vi "Apply VNS to Random Solution.vi"(7 "Max Allowed Time Passed?":bool, 8 "error in (no error)":errorcluster, 10 "GA in":refnum<class "GA.lvclass">, 11 "OSSP_Problem in":refnum<class "OSSP_Problem.lvclass">) -> (0 "error out":errorcluster, 2 "GA out":refnum<class "GA.lvclass">, 3 "OSSP_Problem out":refnum<class "OSSP_Problem.lvclass">)   [LabVIEW 2013]
uses:
  Classes/GA.lvclass
  Classes/OSSP_Problem.lvclass
  Classes/GA.lvclass/GA.ctl
  Classes/OSSP_Problem.lvclass/OSSP_Problem.ctl
  Classes/GA_Class/Controls/Solution_GA.ctl
  Insert Neighborhood.vi
  Inversion Neighborhood.vi
  Zobolas Local Search Engine.vi
  Classes/OSSP_Problem_Class/Getters/Read Number of Machines.vi
  VNS Zobolas LSA Scheduler Selector.vi
  GA/SubVIS/Remove Duplicates In Array.vi
  Generate Two Indices for Local Search.vi
  Or-Opt(Zobolas) Neighborhood.vi
  Swap Neighborhood.vi
  Classes/Scheduler_Class/Prins FIFO Scheduler Methods and Controls/Methods/Calculate Makespan (Prins FIFO Engine).vi
  Classes/Scheduler_Class/Prins FIFO Scheduler Methods and Controls/Methods/Calculate Tardiness (Prins FIFO Engine).vi
  Classes/Scheduler_Class/NonDelay Scheduler/Non Delay Scheduler Engine.vi
  Classes/OSSP_Problem_Class/Getters/Read Number of Jobs.vi
  Classes/OSSP_Problem_Class/Getters/Read Processing Times.vi
  GA/SubVIS/Calcualte General Tardiness.vi
  Classes/OSSP_Problem_Class/Getters/Read Due Dates.vi
  Classes/Scheduler_Class/Giffler Thompson Active Schedule Engine.vi
  Classes/Scheduler_Class/Prins FIFO Scheduler Methods and Controls/Prins FIFO Scheduler.vi
  Classes/Scheduler_Class/Prins FIFO Scheduler Methods and Controls/Methods/Calculate Final Completion Times of Jobs.vi
  Classes/Scheduler_Class/Prins FIFO Scheduler Methods and Controls/Methods/Reorder Schedule(Prins FIFO) based on Start Times.vi
  Classes/Scheduler_Class/Operation to Machine Job Tuple.vi
  Classes/Scheduler_Class/Prins FIFO Scheduler Methods and Controls/Methods/UpdateMachineGaps.vi
  Classes/Scheduler_Class/Prins FIFO Scheduler Methods and Controls/Methods/UpdateJobGaps.vi
  Classes/Scheduler_Class/Prins FIFO Scheduler Methods and Controls/Methods/Find Intersecting Gaps.vi
  Classes/Scheduler_Class/GT Algorithm Find M_ok and J_ok.vi
  Classes/Scheduler_Class/Prins FIFO Scheduler Methods and Controls/Methods/Transform to Plain Job and Machine Gaps Array.vi
  Classes/Scheduler_Class/Semiactive Scheduler/Semi Active Scheduler Engine.vi
  Nonredundant Swap Neighborhood.vi
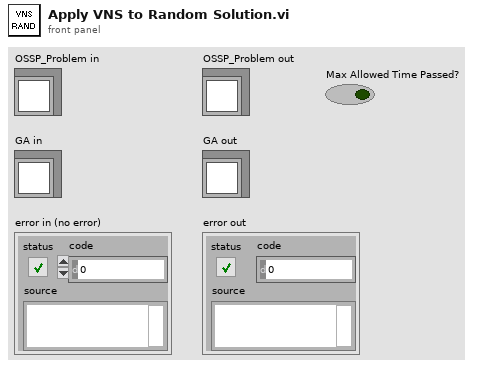
[diagram p1: front panel]
types:
  T1 = typedef "Solution_GA.ctl" = cluster{"Schedule":u16[], "Fitness":u16, "Fitness Valid?":bool}
  T2 = typedef "Objective.ctl" = enum16{"Makespan", "Total Tardiness"}
  T3 = typedef "Scheduler Type.ctl" = enum16{"Non Delay Scheduler", "GT Active Scheduler", "My Faulty Scheduler", "Prins FIFO Scheduler", "SemiActive Scheduler"}
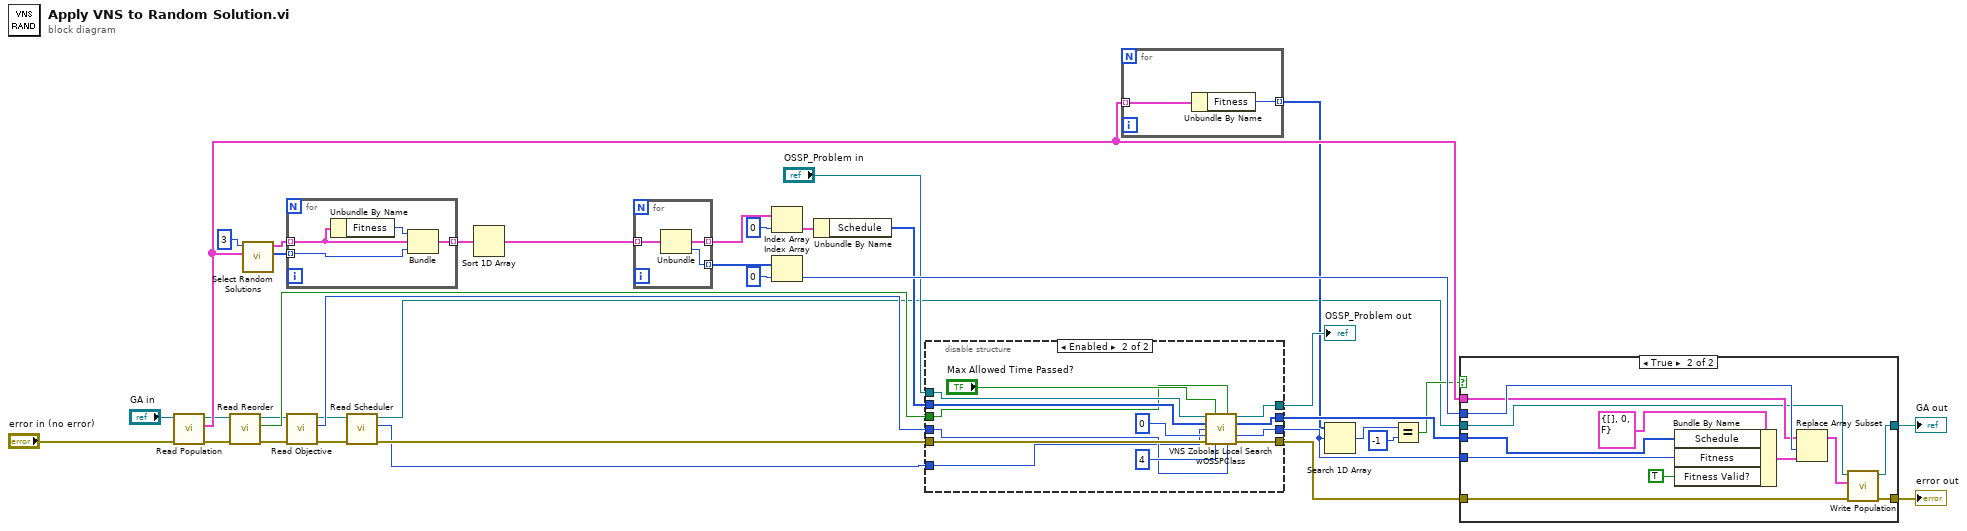
[diagram p0: block diagram]
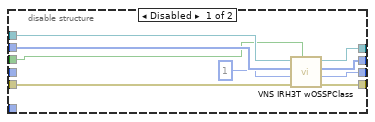
[diagram p3: hidden frame]
diagram:
  n1 = call "Read Population.vi"("error in (no error)"="error in (no error)", "GA in"="GA in") -> ("error out"=w12:errorcluster, "Population"=w20:T1[], "GA out"=w11:refnum<class "GA.lvclass">)  [unwired: 7 in]
  n2 = call "Read Reorder.vi"("error in (no error)"=w12, "GA in"=w11) -> ("error out"=w8:errorcluster, "Reorder"=w10:bool, "GA out"=w7:refnum<class "GA.lvclass">)  [unwired: 7 in]
  n3 = call "Select Random Solutions.vi"("Population"=w20, "Tournament Size"=3) -> ("Solution Indices"=w27:i32[], "Selected Solutions"=w31:T1[])  [unwired: 8 in]
  n4 = for {
    tunnel: w31 -> [w40] mode=indexing
    tunnel: [w39] -> w30 mode=indexing
    tunnel: w27 -> [w38] mode=indexing
    n5 = Unbundle By Name(w40) -> ("Fitness"=w41:u16)
    n6 = Bundle("Fitness"=w41, "Solution"=w40, w38) -> (w39:cluster{"Fitness":u16, "Solution":T1, i32})  [unwired: 1 in]
  }
  n7 = call "Read Objective .vi"("error in (no error)"=w8, "GA in"=w7) -> ("error out"=w3:errorcluster, "Objective"=w6:T2, "GA out"=w5:refnum<class "GA.lvclass">)  [unwired: 7 in]
  n8 = call "Read Scheduler.vi"("error in (no error)"=w3, "GA in"=w5) -> ("error out"=w2:errorcluster, "Scheduler"=w1:T3, "GA out"=w4:refnum<class "GA.lvclass">)  [unwired: 7 in]
  n9 = Sort 1D Array(array=w30) -> (sorted array=w21:cluster{"Fitness":u16, "Solution":T1, i32}[])
  n10 = for {
    tunnel: w21 -> [w44] mode=indexing
    tunnel: [w43] -> w29 mode=indexing
    tunnel: [w42] -> w26 mode=indexing
    n11 = Unbundle(w44) -> ("Solution"=w43:T1, w42:i32)  [unwired: 1 out]
  }
  n12 = Index Array(array=w29, index=0) -> (element=w24:T1)
  n13 = Index Array(array=w26, index=0) -> (element=w22:i32)
  n14 = Unbundle By Name(w24) -> ("Schedule"=w15:u16[])
  n15 = disable-structure shown="Enabled" {
    disable-tunnel: [w53 w65] -> w33
    disable-tunnel: [w52 w59] -> w23
    disable-tunnel: [w51 w61] -> w17
    disable-tunnel: [w50 w62] -> w16
    disable-tunnel: w15 -> [w49 w64]
    disable-tunnel: "OSSP_Problem in" -> [w48 w66]
    disable-tunnel: w2 -> [w46 w60]
    disable-tunnel: w10 -> [w45 w56]
    disable-tunnel: w6 -> [_ w55]
    disable-tunnel: w1 -> [_ w54]
    frame Disabled {
      n16 = call "VNS IRH3T wOSSPClass.vi"("Reorder?"=w45, "error in (no error)"=w46, "Max Iteration Count"=1, "Best Chromosome In"=w49, "OSSP_Problem.lvclass"=w48) -> ("error out"=w52:errorcluster, "Tardiness(FIFO Engine)"=w51:u16, "VNS Result"=w50:u16[], "OSSP_Problem out"=w53:refnum<class "OSSP_Problem.lvclass">)  [unwired: 3 in]
    }
    frame Enabled {
      n17 = call "VNS Zobolas Local Search wOSSPClass.vi"("OSSP_Problem.lvclass"=w66, "Max Allowed Time Passed?"="Max Allowed Time Passed?", "Reorder?"=w56, "Schedule In"=w64, "Scheduler"=w54, "Max Iteration Count"=0, "error in (no error)"=w60, "Number of Neighborhoods"=4, "Objective"=w55) -> ("OSSP_Problem out"=w65:refnum<class "OSSP_Problem.lvclass">, "VNS Result Out"=w62:u16[], "Makespan/Tardiness(FIFO Engine)"=w61:u16, "error out"=w59:errorcluster)  [unwired: 3 in]
    }
  }
  "OSSP_Problem out" <- w33
  n18 = for {
    tunnel: w20 -> [w68] mode=indexing
    tunnel: [w67] -> w13 mode=indexing
    n19 = Unbundle By Name(w68) -> ("Fitness"=w67:u16)
  }
  n20 = Search 1D Array(1D array=w13, element=w17) -> (index of element=w19:i32)  [unwired: 1 in]
  n21 = Equal?(x=w19, y=-1) -> (x = y?=w9:bool)
  n22 = case shown="True" w9 {
    tunnel: [w70 w82] -> w37
    tunnel: [w69 w81] -> w36
    tunnel: w23 -> [w69 w80]
    tunnel: w22 -> [_ w79]
    tunnel: w20 -> [_ w78]
    tunnel: w17 -> [_ w77]
    tunnel: w16 -> [_ w76]
    tunnel: w4 -> [w70 w75]
    frame False {
    }
    frame True {
      n23 = Bundle By Name(cluster=T1 {"Schedule"=[], "Fitness"=0, "Fitness Valid?"=FALSE} ("Solution"), "Schedule"=w76, "Fitness"=w77, "Fitness Valid?"=TRUE) -> (w72:T1)
      n24 = Replace Array Subset(array=w78, new element=w72, index=w79) -> (w71:T1[])
      n25 = call "Write Population.vi"("error in (no error)"=w80, "Population"=w71, "GA in"=w75) -> ("error out"=w81:errorcluster, "GA out"=w82:refnum<class "GA.lvclass">)  [unwired: 7 in]
    }
  }
  "GA out" <- w37
  "error out" <- w36
